vi "Return_Gauge_RP_SubVi.vi"(10 "number":dbl, 11 "Knob in":refnum<vi>) -> (3 "Gauge":dbl(knob) scale=0.0..8.0)   [LabVIEW 2014]
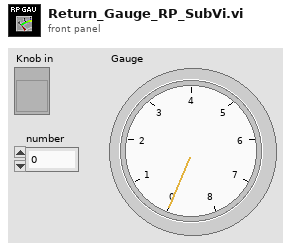
[diagram p1: front panel]
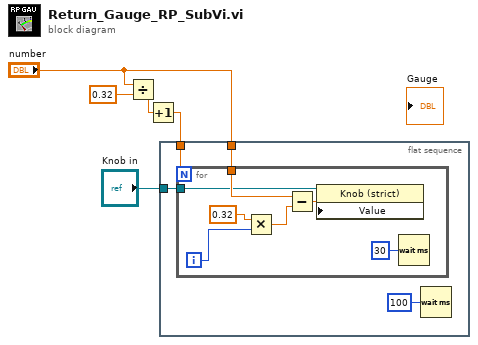
[diagram p0: block diagram]
diagram:
  n1 = Divide(x="number", y=0.32) -> (x/y=w4:dbl)
  n2 = Increment(x=w4) -> (x+1=w5:dbl)
  n3 = flat-sequence {
    tunnel: w5 -> [w8]
    tunnel: "number" -> [w7]
    tunnel: "Knob in" -> [w6]
    frame #0 {
      n4 = for {
        N: w8 -> [_]
        tunnel: w7 -> [w12]
        tunnel: w6 -> [w10]
        i -> [w14]
        n5 = Multiply(x=0.32, y=w14) -> (x*y=w15:dbl)
        n6 = Subtract(x=w12, y=w15) -> (x-y=w11:dbl)
        n7 = property class="Knob (strict)"(reference=w10, "Value"=w11) -> ()  [unwired: 1 in, 2 out]
        n8 = Wait (ms)(milliseconds to wait=u32 30) -> ()  [unwired: 1 out]
      }
      n9 = Wait (ms)(milliseconds to wait=u32 100) -> ()  [unwired: 1 out]
    }
  }
